vi "Insert Channel at Index.vi"(8 "error in (no error)":errorcluster, 9 "Channel":refnum<class "Configuration.Channel.lvclass">, 10 "index":i32, 11 "Transfer Configuration in":refnum<class "Configuration.Transfer.lvclass">) -> (0 "error out":errorcluster, 3 "Transfer Configuration out":refnum<class "Configuration.Transfer.lvclass">)   [LabVIEW 2016, in "Configuration.Transfer.lvclass"]
uses:
  Configuration.Transfer.lvclass
  Configuration.Channel/Configuration.Channel.lvclass
  Configuration.Transfer.lvclass/Configuration.Transfer.ctl
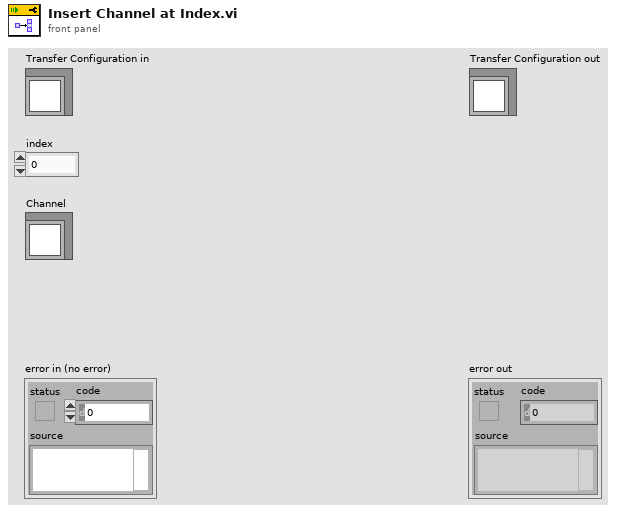
[diagram p1: front panel]
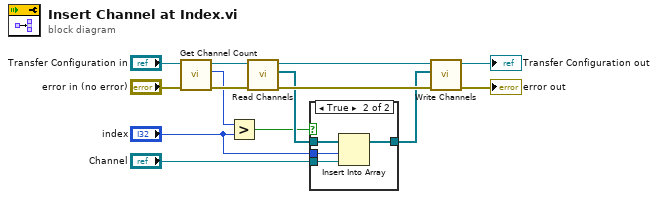
[diagram p0: block diagram]
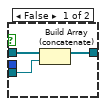
[diagram p2: hidden frame]
diagram:
  n1 = call "Get Channel Count.vi"("error in (no error)"="error in (no error)", "Transfer Configuration in"="Transfer Configuration in") -> ("error out"=w5:errorcluster, "channel count"=w4:i32, "Transfer Configuration out"=w6:refnum<class "Configuration.Transfer.lvclass">)  [unwired: 7 in]
  n2 = Greater?(x=w4, y="index") -> (0:w2:bool)
  n3 = call "Read Channels.vi"("error in (no error)"=w5, "Configuration.Transfer in"=w6) -> ("error out"=w13:errorcluster, "Channels"=w10:refnum<class "Configuration.Channel.lvclass">[], "Configuration.Transfer out"=w14:refnum<class "Configuration.Transfer.lvclass">)  [unwired: 7 in]
  n4 = case shown="True" w2 {
    tunnel: w10 -> [w17 w21]
    tunnel: [w15 w20] -> w1
    tunnel: "Channel" -> [w16 w19]
    tunnel: "index" -> [_ w18]
    frame False {
      n5 = Build Array (concatenate)(w17, w16) -> (w15:refnum<class "Configuration.Channel.lvclass">[])
    }
    frame True {
      n6 = Insert Into Array(array=w21, index=w18, new element=w19) -> (w20:refnum<class "Configuration.Channel.lvclass">[])
    }
  }
  n7 = call "Write Channels.vi"("error in (no error)"=w13, "Channels"=w1, "Configuration.Transfer in"=w14) -> ("error out"=→"error out":errorcluster, "Configuration.Transfer out"=→"Transfer Configuration out":refnum<class "Configuration.Transfer.lvclass">)  [unwired: 7 in]
